vi "BGSub.vi"(7 "index":i32, 8 "error in (no error)":errorcluster, 10 "BG IN":T1, 11 "raw Image In":T1) -> (0 "error out":errorcluster, 3 "Refnum out":T1, 4 "empty image":bool)   [LabVIEW 2013]
uses:
  <vilib>/vision/Image Controls.llb/IMAQ Image.ctl
  <vilib>/vision/NI_Vision_Development_Module.lvlib
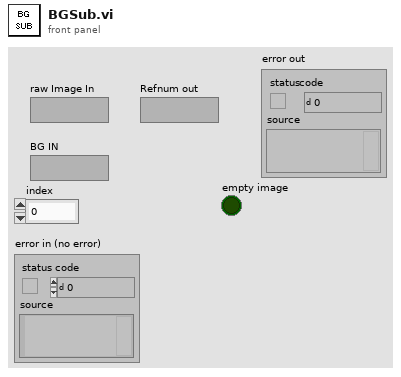
[diagram p1: front panel]
types:
  T1 = typedef "IMAQ Image.ctl" = refnum<image>
  T2 = typedef "Image Type" = u32
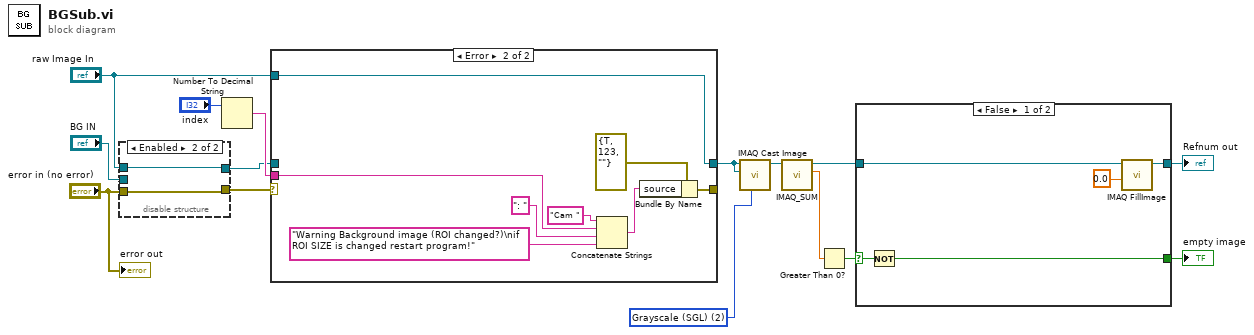
[diagram p0: block diagram]
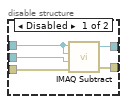
[diagram p2: hidden frame]
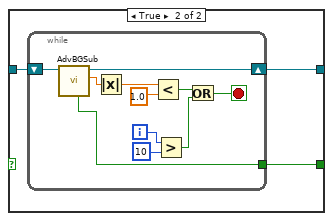
[diagram p4: hidden frame]
diagram:
  w11 = T2 2 items=["Grayscale (U8)", "Grayscale (I16)", "Grayscale (SGL)", "Complex (CSG)", "RGB (U32)", "HSL (U32)", "RGB (U64)", "Grayscale (U16)"] ("Image Type")
  n1 = disable-structure shown="Enabled" {
    disable-tunnel: "BG IN" -> [w20 _]
    disable-tunnel: [w19 w21] -> w8
    disable-tunnel: "raw Image In" -> [w18 w22]
    disable-tunnel: [w17 w22] -> w3
    disable-tunnel: "error in (no error)" -> [w16 w21]
    frame Disabled {
      n2 = call "IMAQ Subtract"("Image Src A"=w18, "Image Dst"=w18, "Image Src B"=w20, "error in (no error)"=w16) -> ("Image Dst Out"=w17:T1, "error out"=w19:errorcluster)  [unwired: 3 in]
    }
    frame Enabled {
    }
  }
  n3 = Number To Decimal String(number="index") -> (decimal integer string=w6:string)  [unwired: 1 in]
  n4 = case shown="Error" w8 {
    selector: w8 -> [w24 _]
    tunnel: [w24 w26] -> _
    tunnel: w6 -> [_ w31]
    tunnel: "raw Image In" -> [_ w25]
    tunnel: [w23 w25] -> w2
    tunnel: w3 -> [w23 _]
    frame No Error {
    }
    frame Error {
      n5 = Concatenate Strings("Cam " ("string"), w31, ": " ("string"), "Warning Background image (ROI changed?)\nif ROI SIZE is changed restart program!" ("source")) -> (w27:string)
      n6 = Bundle By Name(cluster=errorcluster {"status"=TRUE, "code"=123, "source"=""} ("error out"), "source"=w27) -> (w26:errorcluster)
    }
  }
  n7 = call "IMAQ Cast Image"("Image Type"=w11, "Image Dst"=w2, "Image Src"=w2) -> ("Image Dst Out"=w12:T1)  [unwired: 7 in, 1 out]
  n8 = call "IMAQ_SUM.vi"("Image"=w12) -> ("Sum"=w13:sgl, "Image 2"=w14:T1)  [unwired: 9 in]
  n9 = Greater Than 0?(x=w13) -> (x > 0?=w15:bool)
  n10 = case shown="False" w15 {
    selector: w15 -> [w34 _]
    tunnel: [w35 w40] -> w10
    tunnel: w14 -> [w37 w39]
    tunnel: [w33 w38] -> w7
    frame False {
      n11 = Not(x=w34) -> (.not. x?=w33:bool)
      n12 = call "IMAQ FillImage"("Pixel Value (U8, U16, I16, Float)"=sgl 0.0, "Image"=w37) -> ("Image Out"=w35:T1)  [unwired: 8 in, 1 out]
    }
    frame True {
      n13 = while {
        shift-right: [w51] -> w40
        shift-left: w39 -> [w50]
        tunnel: [w41] -> w38
        i -> [w49]
        stop <- w48 stop-if-true
        n14 = call "AdvBGSub.vi"("Refnum in"=w50) -> ("-x"=w43:sgl, "Refnum out"=w51:T1, "empty image"=w41:bool)  [unwired: 7 in, 1 out]
        n15 = Absolute Value(x=w43) -> (abs(x)=w42:sgl)
        n16 = Less?(x=w42, y=sgl 1.0) -> (x < y?=w46:bool)
        n17 = Greater?(x=w49, y=10) -> (0:w44:bool)
        n18 = Or(x=w46, y=w44) -> (x .or. y?=w48:bool)
      }
    }
  }
  "Refnum out" <- w10
  "empty image" <- w7
  "error out" <- "error in (no error)"
